vi "Host - Get Slaves.vi"(8 "error in (no error)":errorcluster, 11 "Master Ref in":refnum<k21>) -> (0 "error out":errorcluster, 2 "Slaves":T1[](array[typedef]), 3 "Master Ref out":refnum<k21>)   [LabVIEW 2016, in "Scan Engine Custom Device.lvlib"]
uses:
  Scan Engine Custom Device.lvlib
  Type Defs/Host - Slave.ctl
  Type Defs/Host - Module.ctl
  <resource>/objmgr/IndComECAT.rc
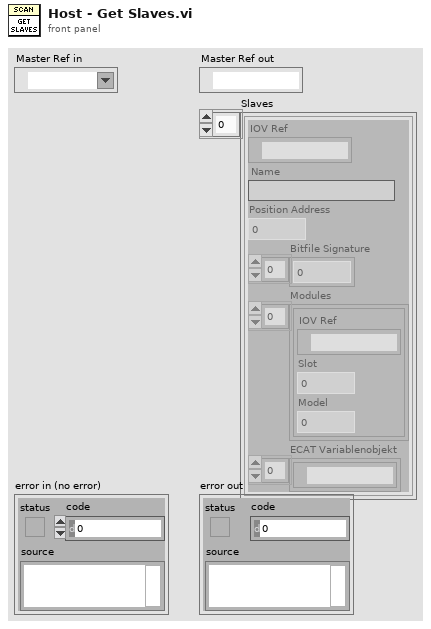
[diagram p1: front panel]
types:
  T1 = typedef "Scan Engine Custom Device.lvlib/Host - Slave.ctl" = cluster{"IOV Ref":refnum<k21>, "Name":string, "Position Address":u16, "Bitfile Signature":u8[], "Modules":T2[], "ECAT Variablenobjekt":refnum<k21>[]}
  T2 = typedef "Scan Engine Custom Device.lvlib/Host - Module.ctl" = cluster{"IOV Ref":refnum<k21>, "Slot":u32, "Model":u32}
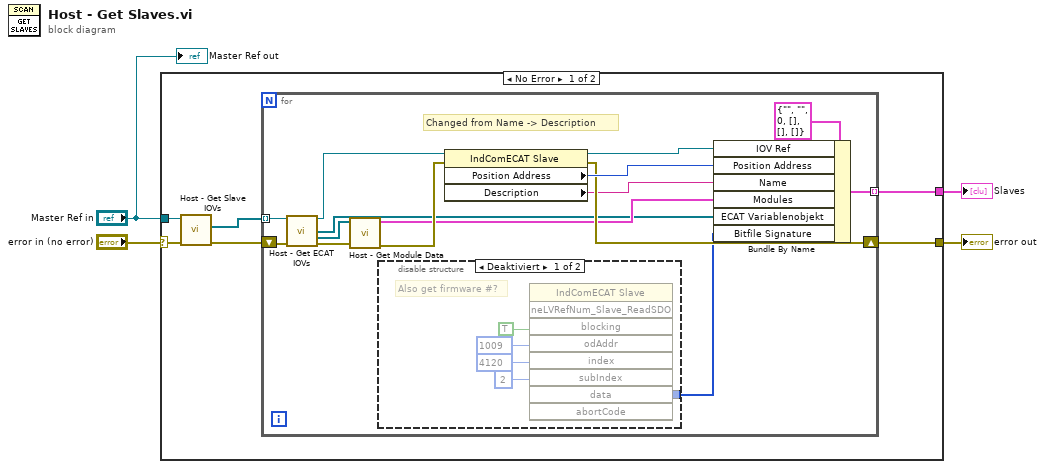
[diagram p0: block diagram]
diagram:
  n1 = case shown="No Error" "error in (no error)" {
    selector: "error in (no error)" -> [w5 w31]
    tunnel: [w10 _] -> w4
    tunnel: [w9 w31] -> w3
    tunnel: "Master Ref in" -> [w8 _]
    frame No Error {
      n2 = call "Host - Get Slave IOVs.vi"("error in (no error)"=w5, "ECAT Master in"=w8) -> ("error IO"=w7:errorcluster, "All Slaves"=w6:refnum<k21>[])  [unwired: 7 in, 1 out]
      n3 = for {
        tunnel: w6 -> [w22] mode=indexing
        tunnel: [w16] -> w10 mode=indexing
        shift-right: [w15] -> w9
        shift-left: w7 -> [w23]
        # "Changed from Name -> Description"
        n4 = call "Host - Get ECAT IOVs.vi"("ECAT Slave in"=w22, "error in (no error)"=w23) -> ("ECAT Slave out"=w21:refnum<k21>, "ECAT Variablenobjekt"=w11:refnum<k21>[], "All Mods"=w25:refnum<k21>[], "error IO"=w24:errorcluster)  [unwired: 9 in, 1 out]
        n5 = call "Host - Get Module Data.vi"("error in (no error)"=w24, "Mod IOVs"=w25) -> ("error out"=w20:errorcluster, "Modules"=w13:T2[])  [unwired: 8 in]
        n6 = disable-structure shown="Deaktiviert" {
          disable-tunnel: [w26 _] -> w12
          frame Disabled {
            # "Also get firmware #?"
            n7 = invoke class="IndComECAT Slave" method="neLVRefNum_Slave_ReadSDO"("blocking"=TRUE, "odAddr"=u16 1009, "index"=u16 4120, "subIndex"=u8 2) -> ("data"=w26:u8[])  [unwired: 5 in, 8 out]
          }
          frame Enabled {
          }
        }
        n8 = property class="IndComECAT Slave"(reference=w21, error in=w20) -> (reference out=w18:refnum<k21>, error out=w15:errorcluster, "Position Address"=w17:u16, "Description"=w14:string)
        n9 = Bundle By Name(cluster=T1 {"IOV Ref"="", "Name"="", "Position Address"=0, "Bitfile Signature"=[], "Modules"=[], "ECAT Variablenobjekt"=[]} ("Slave"), "IOV Ref"=w18, "Position Address"=w17, "Name"=w14, "Modules"=w13, "ECAT Variablenobjekt"=w11, "Bitfile Signature"=w12) -> (w16:T1)
      }
    }
    frame Error {
    }
  }
  "Slaves" <- w4
  "error out" <- w3
  "Master Ref out" <- "Master Ref in"
